vi "Initialize System (Single Line).vi"(0 "wiring":T1=enum."3xUph + 4xI", 1 "samples per cycle (192)":u16=192 min=128 max=512, 5 "nominal frequency":enum16{"50 Hz", "60 Hz"}(ring), 7 "nominal voltage (230 V)":dbl=230.0, 9 "type of reference voltage":enum16{"Constant", "Sliding"}(ring), 11 "error in (no error)":errorcluster) -> (4 "nominal sample rate [Hz]":u16, 10 "system info out":refnum<class "EP System Info.lvclass">, 15 "error out":errorcluster)   [LabVIEW 2014, in "NI_EP_Power Quality.lvlib"]
doc: "Sets the basic configuration of the electrical power system based on different line and bus configurations. You must manually select the polymorphic instance you want to use."
uses:
  <vilib>/addons/Electrical Power/PQ/NI_EP_Power Quality.lvlib
  <vilib>/addons/Electrical Power/PQ/Common/Controls/ep_Wiring.ctl
  <vilib>/addons/Electrical Power/PQ/Common/Classes/System Info/EP System Info.lvclass
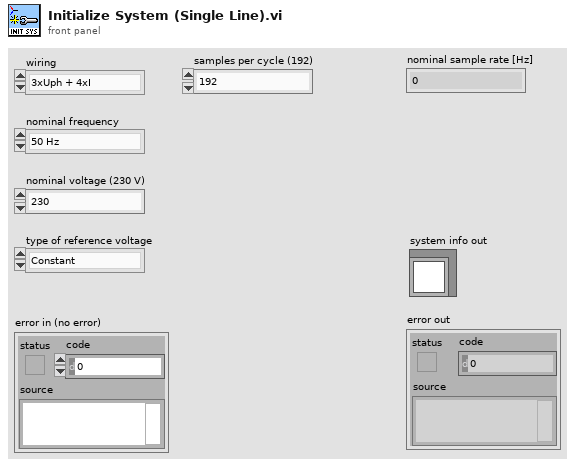
[diagram p1: front panel]
types:
  T1 = typedef "NI_EP_Power Quality.lvlib/ep_Wiring.ctl" = enum16{"4xUph + 4xI", "3xUph + 4xI", "3xUline + 4xI", "3xUph + 3xI", "3xUline + 3xI", "3xUph + 2xI", "3xUline + 2xI", "1xUph + 1xI"}
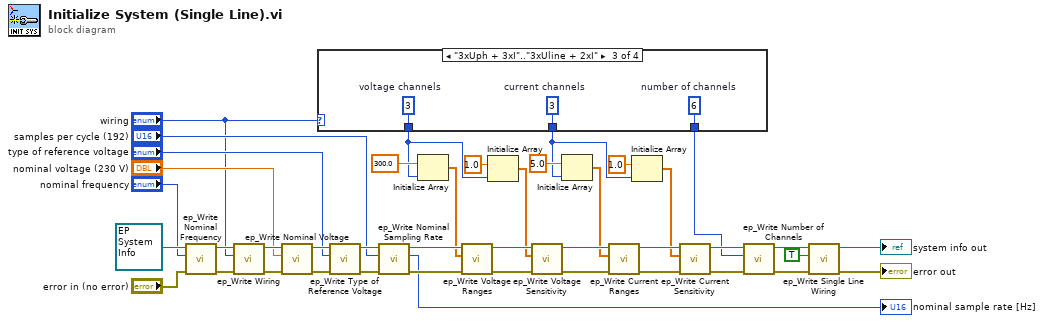
[diagram p0: block diagram]
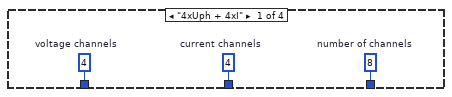
[diagram p2: hidden frame]
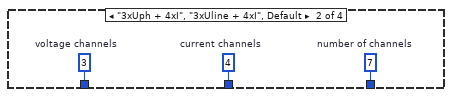
[diagram p3: hidden frame]
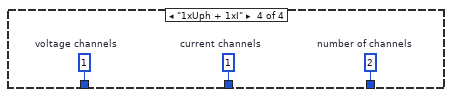
[diagram p4: hidden frame]
diagram:
  n1 = call <vilib>:"ep_Write Nominal Frequency.vi"("error in (no error)"="error in (no error)", "nominal frequency"="nominal frequency", "system info in"=refnum<class "EP System Info.lvclass"> refnum ("EP System Info.lvclass")) -> ("error out"=w39:errorcluster, "system info out"=w40:refnum<class "EP System Info.lvclass">)  [unwired: 7 in]
  n2 = call <vilib>:"ep_Write Wiring.vi"("error in (no error)"=w39, "wiring"="wiring", "system info in"=w40) -> ("error out"=w37:errorcluster, "system info out"=w38:refnum<class "EP System Info.lvclass">)  [unwired: 7 in]
  n3 = call <vilib>:"ep_Write Nominal Voltage.vi"("error in (no error)"=w37, "nominal voltage [V]"="nominal voltage (230 V)", "system info in"=w38) -> ("error out"=w35:errorcluster, "system info out"=w36:refnum<class "EP System Info.lvclass">)  [unwired: 7 in]
  n4 = case shown="\"3xUph + 3xI\"..\"3xUline + 2xI\"" "wiring" {
    tunnel: [w45 w48 w51 w54] -> w16
    tunnel: [w44 w47 w50 w53] -> w12
    tunnel: [w43 w46 w49 w52] -> w6
    frame "4xUph + 4xI" {
      w43 = 8  # number of channels
      w44 = 4  # current channels
      w45 = 4  # voltage channels
    }
    frame "3xUph + 4xI", "3xUline + 4xI", Default {
      w46 = 7  # number of channels
      w47 = 4  # current channels
      w48 = 3  # voltage channels
    }
    frame "3xUph + 3xI".."3xUline + 2xI" {
      w49 = 6  # number of channels
      w50 = 3  # current channels
      w51 = 3  # voltage channels
    }
    frame "1xUph + 1xI" {
      w52 = 2  # number of channels
      w53 = 1  # current channels
      w54 = 1  # voltage channels
    }
  }
  n5 = call <vilib>:"ep_Write Type of Reference Voltage.vi"("error in (no error)"=w35, "type of reference voltage"="type of reference voltage", "system info in"=w36) -> ("error out"=w31:errorcluster, "system info out"=w30:refnum<class "EP System Info.lvclass">)  [unwired: 7 in]
  n6 = call <vilib>:"ep_Write Nominal Sampling Rate.vi"("error in (no error)"=w31, "samples per cycle"="samples per cycle (192)", "system info in"=w30) -> ("error out"=w23:errorcluster, "nominal sampling rate [Hz]"=→"nominal sample rate [Hz]":u16, "system info out"=w19:refnum<class "EP System Info.lvclass">)  [unwired: 6 in]
  n7 = Initialize Array(300.0, w16) -> (w18:dbl[])
  n8 = call <vilib>:"ep_Write Voltage Ranges.vi"("error in (no error)"=w23, "voltage ranges"=w18, "system info in"=w19) -> ("error out"=w26:errorcluster, "system info out"=w22:refnum<class "EP System Info.lvclass">)  [unwired: 7 in]
  n9 = Initialize Array(1.0, w16) -> (w15:dbl[])
  n10 = call <vilib>:"ep_Write Voltage Sensitivity.vi"("error in (no error)"=w26, "voltage sensitivity"=w15, "system info in"=w22) -> ("error out"=w25:errorcluster, "system info out"=w21:refnum<class "EP System Info.lvclass">)  [unwired: 7 in]
  n11 = Initialize Array(5.0, w12) -> (w11:dbl[])
  n12 = call <vilib>:"ep_Write Current Ranges.vi"("error in (no error)"=w25, "current ranges"=w11, "system info in"=w21) -> ("error out"=w24:errorcluster, "system info out"=w20:refnum<class "EP System Info.lvclass">)  [unwired: 7 in]
  n13 = Initialize Array(1.0, w12) -> (w10:dbl[])
  n14 = call <vilib>:"ep_Write Current Sensitivity.vi"("error in (no error)"=w24, "current sensitivity"=w10, "system info in"=w20) -> ("error out"=w7:errorcluster, "system info out"=w8:refnum<class "EP System Info.lvclass">)  [unwired: 7 in]
  n15 = call <vilib>:"ep_Write Number of Channels.vi"("error in (no error)"=w7, "number of channels"=w6, "system info in"=w8) -> ("error out"=w4:errorcluster, "system info out"=w5:refnum<class "EP System Info.lvclass">)  [unwired: 7 in]
  n16 = call <vilib>:"ep_Write Single Line Wiring.vi"("error in (no error)"=w4, "single line wiring? (F)"=TRUE, "system info in"=w5) -> ("error out"=→"error out":errorcluster, "system info out"=→"system info out":refnum<class "EP System Info.lvclass">)  [unwired: 7 in]
